vi "03 - Simple HTTP Data Connection.vi"() -> ()   [LabVIEW 2021]
uses:
  <vilib>/JDP Science/JSONtext/LVClass Serializer/JSONtext LVClass Serializer.lvclass
  7801d39f-66b7-4e88-ad6f-c875adc63ad7.vi
  <vilib>/httpClient/LabVIEWHTTPClient.lvlib
panel:
  in  "Stop":bool
  out "userId data":T1(array[cluster])
  out "body 3":string
  in  "record id":i32=1
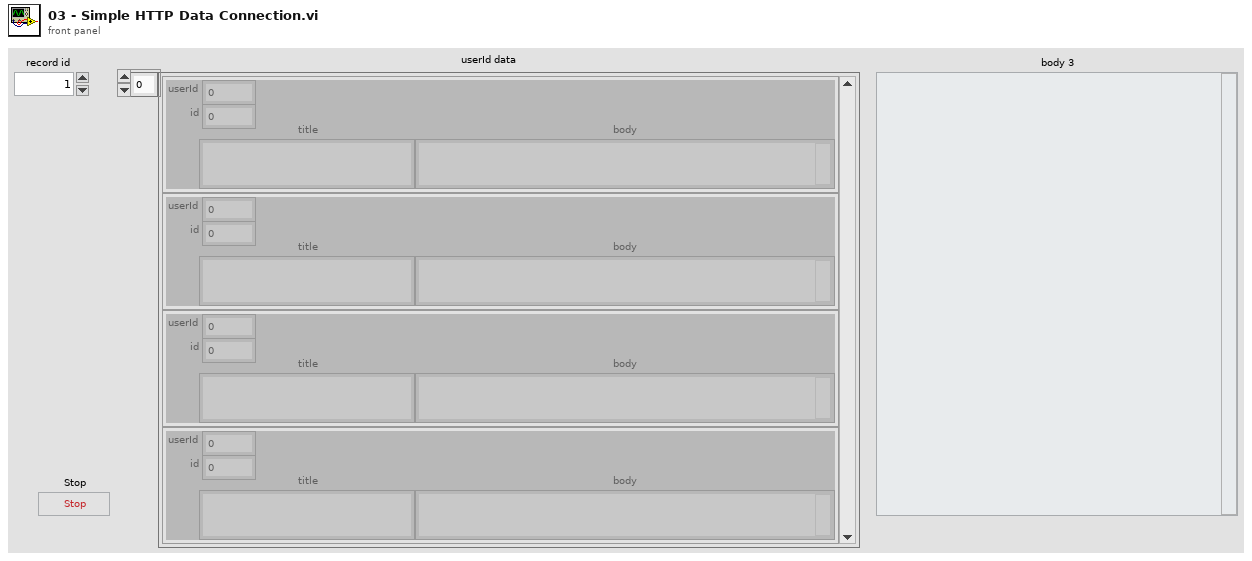
[diagram p1: front panel]
types:
  T1 = cluster{"userId":dbl, "id":dbl, "title":string, "body":string}[]
  T2 = typedef "LabVIEWHTTPClient.lvlib/ClientHandle.ctl" = refnum<k1>
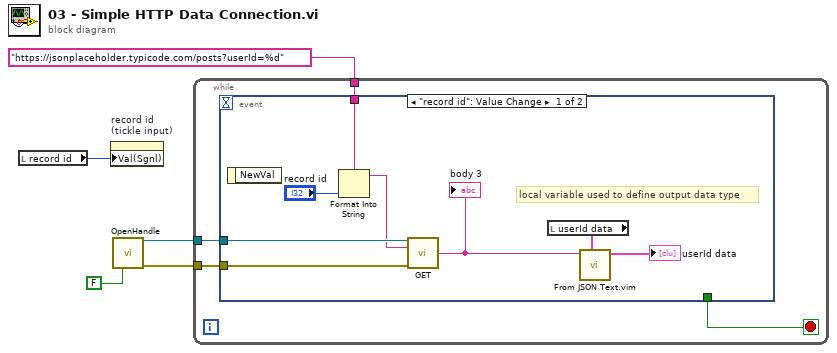
[diagram p0: block diagram]
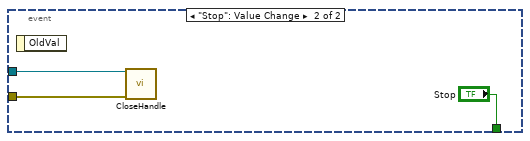
[diagram p2: hidden frame]
diagram:
  n1 = local read "record id"() -> (w2:i32)
  n2 = property on="record id\n(tickle input)" class="DigNum (strict)"("Val(Sgnl)"=w2) -> ()  [unwired: 2 in, 2 out]
  n3 = call <vilib>:"OpenHandle.vi"("verify server(true)"=FALSE ("verify server (T)")) -> ("client handle out"=w3:T2, "error out"=w5:errorcluster)  [unwired: 13 in]
  n4 = while {
    tunnel: w3 -> [w8]
    tunnel: w5 -> [w9]
    tunnel: "https://jsonplaceholder.typicode.com/posts?userId=%d" ("url") -> [w7]
    stop <- w6 stop-if-true
    n5 = event shown="[0] \"record id\": Value Change" {
      selector: _ -> [_ _]
      dyn-events: _ -> [_ _]
      timeout: _ -> [_ _]
      tunnel: w8 -> [w16 w18]
      tunnel: w9 -> [w17 w19]
      tunnel: w7 -> [w10 _]
      tunnel: [_ "Stop"] -> w6
      event "record id": Value Change {
        # "local variable used to define output data type"
        n6 = event-data() -> ()  [unwired: 1 in, 1 out]
        n7 = Format Into String(format string=w10, "record id") -> (resulting string=w15:string)  [unwired: 2 in, 1 out]
        n8 = call <vilib>:"GET.vi"("client handle"=w16, "url"=w15, "error in (no error)"=w17) -> ("body"=w13:string)  [unwired: 9 in, 3 out]
        "body 3" <- w13
        n9 = local read "userId data"() -> (w12:T1)
        n10 = call "From JSON Text.vim"("Data Type and Default Value"=w12, "JSON"=w13) -> ("Data out"=→"userId data":T1)  [unwired: 8 in, 1 out]
      }
      event "Stop": Value Change {
        n11 = event-data() -> ()  [unwired: 1 in, 1 out]
        n12 = call <vilib>:"CloseHandle.vi"("client handle"=w18, "error in (no error)"=w19) -> ()  [unwired: 13 in, 1 out]
      }
    }
  }
